vi "generate indexed directories.vi"(10 "image # left in":i32, 11 "path in":path) -> (1 "image # left out":i32, 2 "Imaging State out":T1, 3 "path out":path)   [LabVIEW 2013]
uses:
  Imaging State.ctl
  <vilib>/regexp/Match Regular Expression.xnode
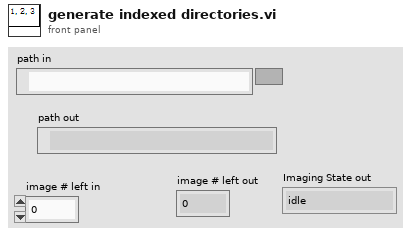
[diagram p1: front panel]
types:
  T1 = typedef "Imaging State.ctl" = enum16{"idle", "waiting for saving sheet", "waiting for stopping", "waiting for saving tiff", "init countinuous saving", "continuous saving", ""}
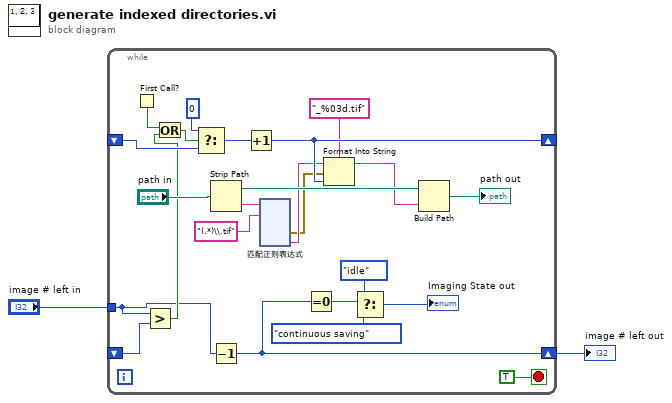
[diagram p0: block diagram]
diagram:
  n1 = while {
    shift-right: [w16] -> _
    shift-left: _ -> [w11]
    shift-right: [w6] -> w1
    shift-left: _ -> [w5]
    tunnel: "image # left in" -> [w3]
    stop <- TRUE stop-if-true
    n2 = First Call?() -> (First Call?: T/F=w8:bool)
    n3 = Greater?(x=w3, y=w5) -> (0:w4:bool)
    n4 = Or(x=w8, y=w4) -> (x .or. y?=w7:bool)
    n5 = Select(t=0, s=w7, f=w11) -> (s? t:f=w10:i32)
    n6 = Strip Path(path="path in") -> (stripped path=w24:path, name=w17:string)
    n7 = Decrement(x=w3) -> (x-1=w6:i32)
    n8 = Increment(x=w10) -> (x+1=w16:i32)
    n9 = xnode "匹配正则表达式"("输入字符串"=w17, "正则表达式"="(.*)\\.tif") -> ("错误输出"=w12:errorcluster, "子匹配 1"=w13:string)  [unwired: 4 in, 4 out]
    n10 = Equal To 0?(x=w6) -> (x = 0?=w23:bool)
    n11 = Format Into String(format string="_%03d.tif" ("格式字符串"), initial string=w13, error in=w12, w16) -> (resulting string=w14:string)  [unwired: 1 out]
    n12 = Select(t=Imaging_State."idle" ("Imaging State out"), s=w23, f=Imaging_State."continuous saving") -> (s? t:f=→"Imaging State out":T1)
    n13 = Build Path(base path=w24, name or relative path=w14) -> (appended path=→"path out":path)
  }
  "image # left out" <- w1
